vi "2Voice.FRAME_WR.vi"(0 "VISA resource name":refnum<visa-resource-name> caption="Serial Port", 1 "timeout (10sec)":u32=1000 caption="超时（10秒）", 5 "baud rate (9600)":u32=9600 caption="波特率(9600)", 7 "写入缓冲区":string, 9 "写入字节数组":u8[](array[numeric]) format="%02x", 11 "error in (no error)":errorcluster caption="错误输入（无错误）", 12 "Send Mode":enum16{"0-发送文本", "1-发送16进制数组"}(ring)) -> (4 "Success?":bool, 10 "HEX字符串":string, 15 "error out":errorcluster caption="错误输出")   [LabVIEW 2012, in "Lib_UEL.ATE.lvlib" / "Lib_2Voice.lvlib"]
uses:
  <vilib>/Instr/_visa.llb/VISA Configure Serial Port (Instr).vi
  Lib_2Voice.lvlib
panel:
  out "读取缓冲区":string
  # "V001 - Initial Version. ~LI.Guang 2011-05-13"
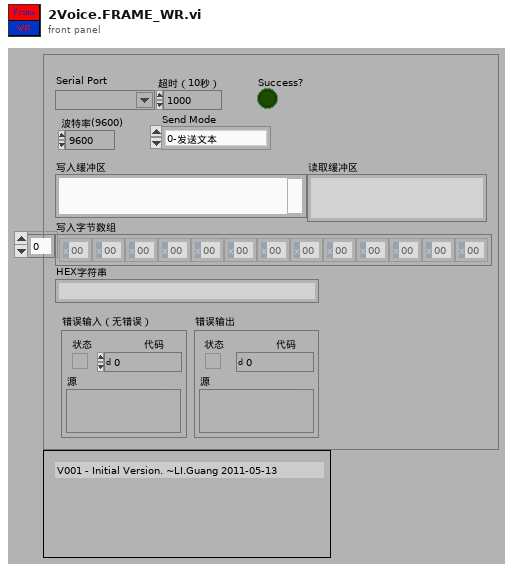
[diagram p1: front panel]
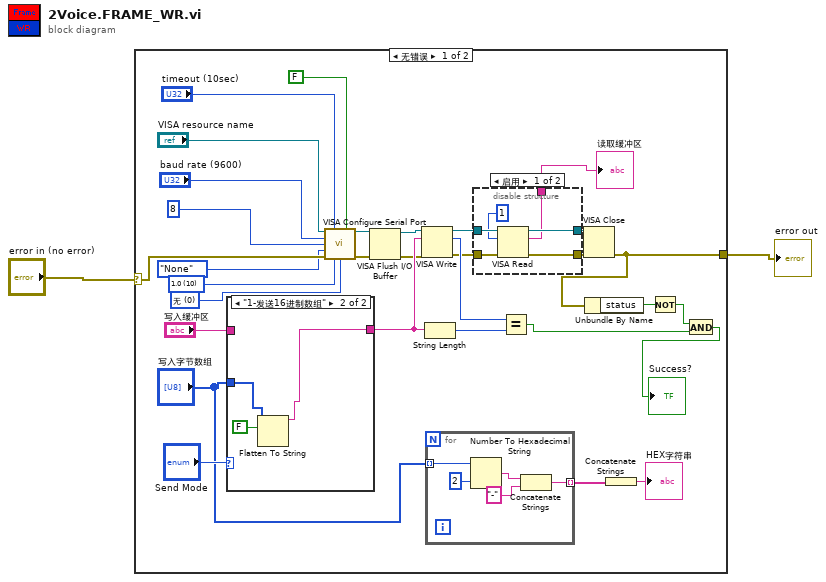
[diagram p0: block diagram]
diagram:
  n1 = case shown="无错误" "error in (no error)" {
    selector: "error in (no error)" -> [w30 w51]
    tunnel: [w25 w51] -> w1
    frame No Error {
      w12 = u16 0 items=["无", "XON/XOFF", "RTS/CTS", "XON/XOFF & RTS/CTS", "DTR/DSR", "XON/XOFF & DTR/DSR"] ("flow control (0:none)")
      w13 = u16 10 items=["1.0"=10, "1.5"=15, "2.0"=20] ("stop bits (10: 1 bit)")
      n2 = case shown="\"1-发送16进制数组\"" "Send Mode" {
        tunnel: "写入字节数组" -> [_ w50]
        tunnel: [w47 w49] -> w21
        tunnel: "写入缓冲区" -> [w47 _]
        frame "0-发送文本", Default {
        }
        frame "1-发送16进制数组" {
          n3 = Flatten To String(anything=w50, prepend array or string size? (T)=FALSE ("预置数组或字符串大小？(T)")) -> (data string=w49:string)  [unwired: 2 in, 2 out]
        }
      }
      n4 = call-poly "VISA Configure Serial Port"("VISA resource name"="VISA resource name", "timeout (10sec)"="timeout (10sec)", "Enable Termination\nChar (T)"=FALSE ("Disable Termination\nChar (T)"), "baud rate (9600)"="baud rate (9600)", "data bits (8)"=u16 8, "parity (0:none)"=enum16{"None", "Odd", "Even", "Mark", "Space"}."None", "error in (no error)"=w30, "stop bits (10: 1 bit)"=w13, "flow control (0:none)"=w12) -> ("VISA resource name out"=w5:refnum<visa-resource-name>, "error out"=w6:errorcluster)  [unwired: 5 in]
      n5 = VISA Flush I/O Buffer(VISA resource name=w5, error in (no error)=w6) -> (VISA resource name out=w4:refnum<visa-resource-name>, error out=w3:errorcluster)  [unwired: 1 in]
      n6 = VISA Write(VISA resource name=w4, write buffer=w21, error in (no error)=w3) -> (VISA resource name out=w11:refnum<visa-resource-name>, return count=w28:u32, error out=w10:errorcluster)
      n7 = String Length(string=w21) -> (length=w29:i32)
      n8 = for {
        tunnel: "写入字节数组" -> [w46] mode=indexing
        tunnel: [w42] -> w18 mode=indexing
        n9 = Number To Hexadecimal String(1:i16 2 ("宽度(-)"), 2:w46) -> (0:w44:string)
        n10 = Concatenate Strings(w44, "-" ("字符串")) -> (w42:string)
      }
      n11 = disable-structure shown="启用" {
        disable-tunnel: w11 -> [w39 w41]
        disable-tunnel: w10 -> [w38 w40]
        disable-tunnel: [w37 w41] -> w9
        disable-tunnel: [w36 w40] -> w8
        disable-tunnel: [w34 _] -> w7
        frame Enabled {
          n12 = VISA Read(VISA resource name=w39, byte count=u32 1 ("字节总数"), error in (no error)=w38) -> (VISA resource name out=w37:refnum<visa-resource-name>, read buffer=w34:string, error out=w36:errorcluster)  [unwired: 1 out]
        }
        frame Disabled {
        }
      }
      "读取缓冲区" <- w7
      n13 = Equal?(x=w28, y=w29) -> (x = y?=w24:bool)
      n14 = VISA Close(VISA resource name=w9, error in (no error)=w8) -> (error out=w25:errorcluster)
      n15 = Unbundle By Name(w25) -> ("status"=w26:bool)
      n16 = Concatenate Strings(w18) -> (→"HEX字符串":string)
      n17 = Not(x=w26) -> (.not. x?=w27:bool)
      n18 = And(x=w27, y=w24) -> (x .and. y?=→"Success?":bool)
    }
    frame Error {
    }
  }
  "error out" <- w1
